vi "File Process VI New.vi"(8 "error in (no error)":errorcluster, 11 "Parsed File Path":path) -> (0 "Error Out":errorcluster, 1 "Total Step":u64, 2 "Switching Times":u32[][](array[numeric]), 3 "Channel Names":string[](array[string]), 4 "Initial States":u16[](array[numeric]), 5 "Channel Number":u16, 7 "GPIB Output":string[](array[string]))   [LabVIEW 2012]
panel:
  out "Time Step":dbl
  out "Total Time":dbl
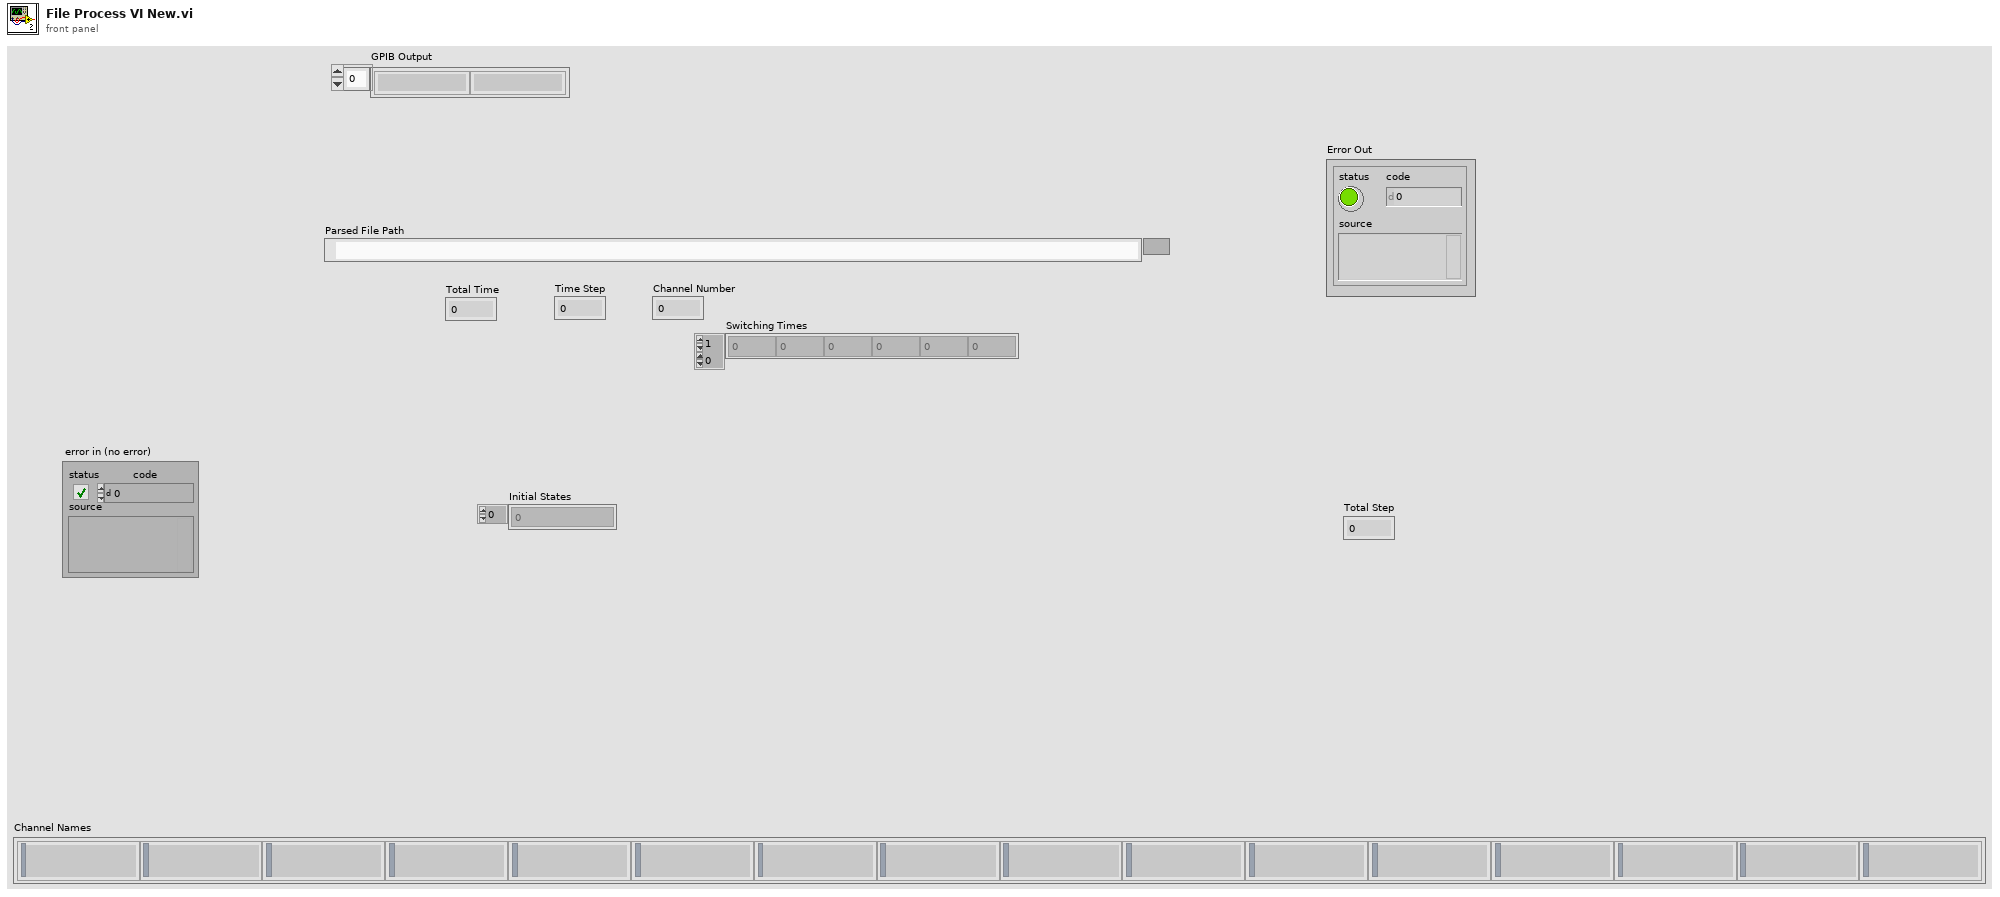
[diagram p1: front panel]
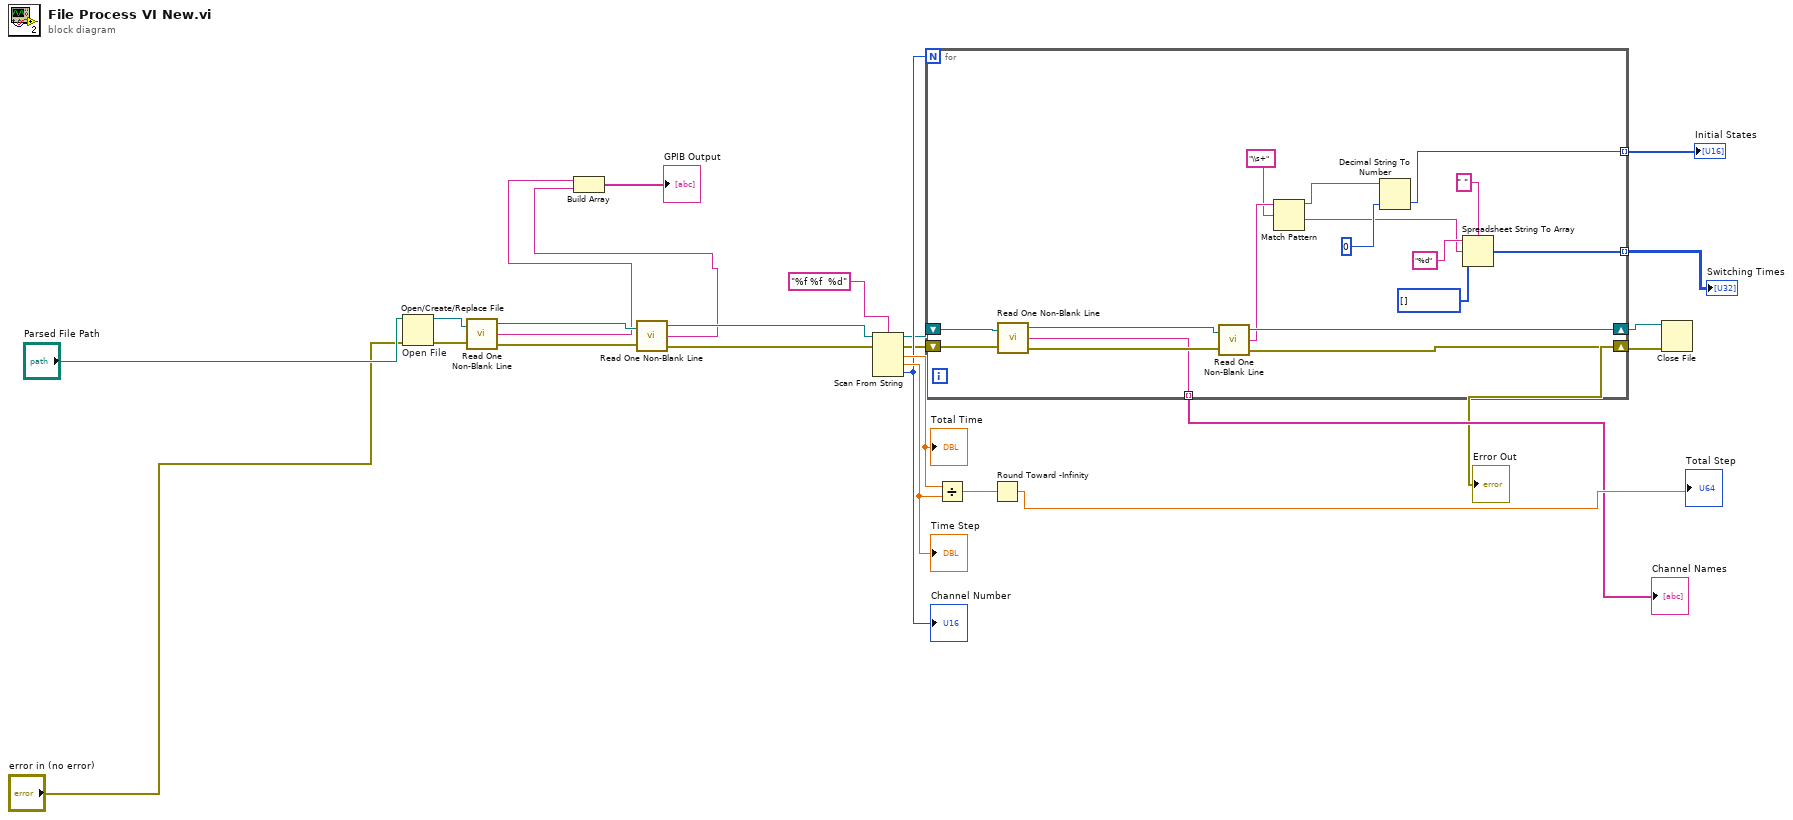
[diagram p0: block diagram]
diagram:
  n1 = Open/Create/Replace File "Open File"(file path (use dialog)="Parsed File Path", error in="error in (no error)") -> (refnum out=w23:refnum<file>, error out=w22:errorcluster)  [unwired: 4 in, 1 out]
  n2 = call "Read One Non-Blank Line.vi"("refnum"=w23, "error in (not an error)"=w22) -> ("dup refnum"=w21:refnum<file>, "Line"=w5:string, "error out"=w19:errorcluster)
  n3 = call "Read One Non-Blank Line.vi"("refnum"=w21, "error in (not an error)"=w19) -> ("dup refnum"=w20:refnum<file>, "Line"=w4:string, "error out"=w18:errorcluster)
  n4 = Build Array(w5, w4) -> (→"GPIB Output":string[])
  n5 = Scan From String("%f %f  %d", w20, w18) -> (w13:refnum<file>, w12:errorcluster, output 1=w17:dbl, output 2=w16:dbl, output 3=w14:u16)  [unwired: 3 in]
  "Total Time" <- w17
  "Time Step" <- w16
  "Channel Number" <- w14
  n6 = for {
    N: w14 -> [_]
    shift-right: [w39] -> w2
    shift-left: w13 -> [w41]
    shift-right: [w36] -> w1
    shift-left: w12 -> [w38]
    tunnel: [w35] -> w9 mode=indexing
    tunnel: [w26] -> w11 mode=indexing
    tunnel: [w25] -> w8 mode=indexing
    n7 = call "Read One Non-Blank Line.vi"("refnum"=w41, "error in (not an error)"=w38) -> ("dup refnum"=w40:refnum<file>, "Line"=w35:string, "error out"=w37:errorcluster)
    n8 = call "Read One Non-Blank Line.vi"("refnum"=w40, "error in (not an error)"=w37) -> ("dup refnum"=w39:refnum<file>, "Line"=w34:string, "error out"=w36:errorcluster)
    n9 = Match Pattern(string=w34, regular expression="\\s+" ("search char (-)")) -> (before substring=w29:string, after substring=w27:string)  [unwired: 1 in, 2 out]
    n10 = Decimal String To Number(string=w29, default (0L)=u16 0) -> (number=w26:u16)  [unwired: 1 in, 1 out]
    n11 = Spreadsheet String To Array(delimiter (Tab)=" ", format string="%d", spreadsheet string=w27, array type (2D Dbl)=u32[] []) -> (array=w25:u32[])
  }
  "Switching Times" <- w8
  "Initial States" <- w11
  "Error Out" <- w1
  "Channel Names" <- w9
  n12 = Divide(x=w17, y=w16) -> (x/y=w15:dbl)
  n13 = Round Toward -Infinity(1:w15) -> (0:→"Total Step":dbl)
  n14 = Close File(refnum=w2, error in=w1) -> ()  [unwired: 2 out]
